vi "hydrolyse_reactor_repetition_check.vi"(10 "#":i32, 11 "Prior Reactor":refnum<vi>) -> (1 "Prior Path":path, 2 "Current Path":path, 3 "Repetition?":bool)   [LabVIEW 2019]
uses:
  lib/libSimulationControl/libSimulationControl.lvlib
panel:
  out "source":path
  out "target":path
  # "*******************************************************************\nBiogas Plant Control\n\nAuthor: Paul Zügel\nGCSC-Frankfurt am Main 2020\n\n*******************************************************************"
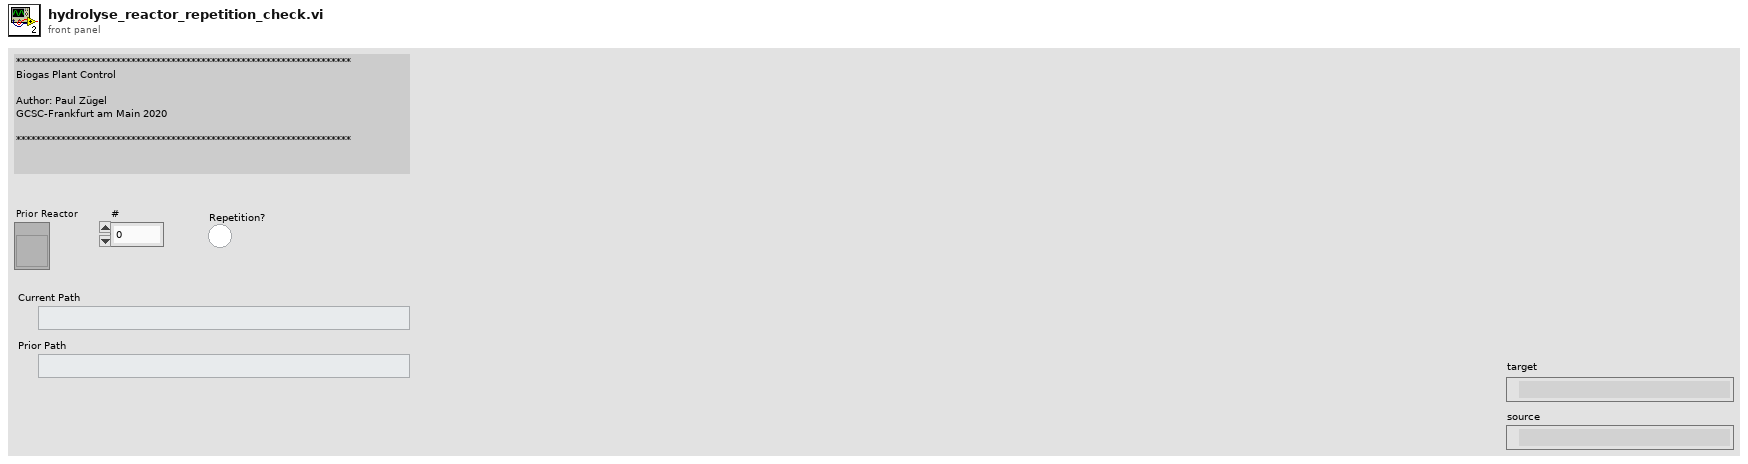
[diagram p1: front panel]
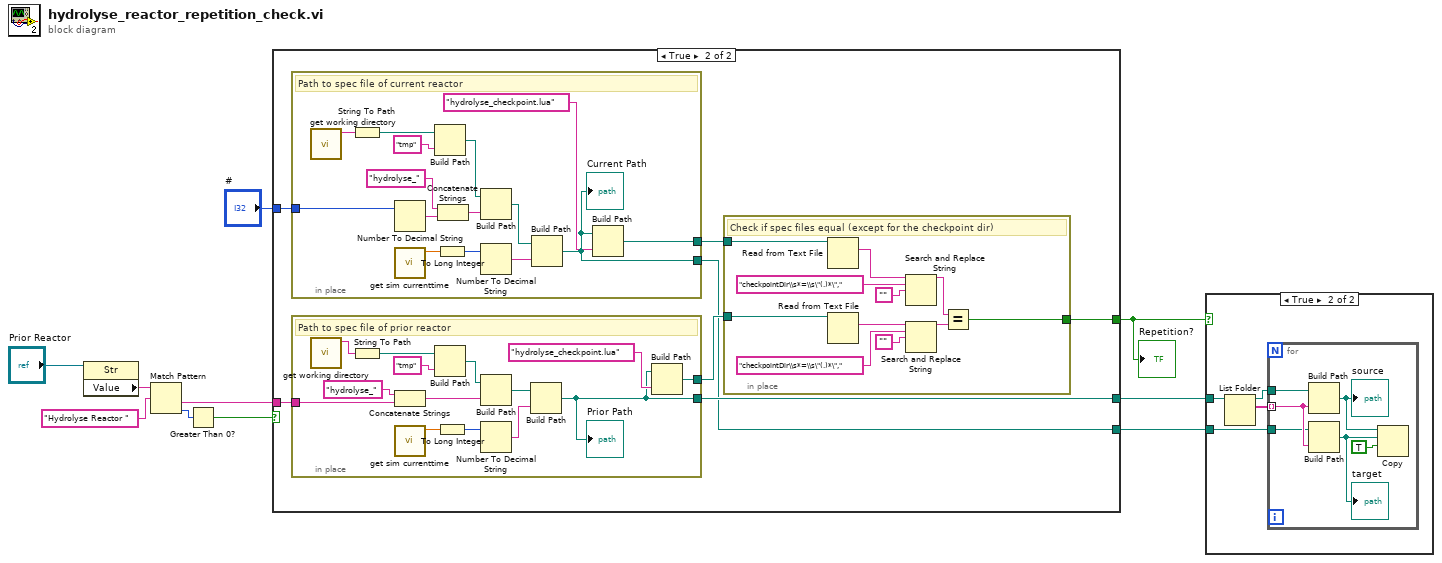
[diagram p0: block diagram]
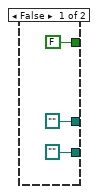
[diagram p3: hidden frame]
diagram:
  n1 = property class="Str"(reference="Prior Reactor") -> ("Value"=w10:string)  [unwired: 1 in, 2 out]
  n2 = Match Pattern(string=w10, regular expression="Hydrolyse Reactor ") -> (after substring=w6:string, offset past match=w8:i32)  [unwired: 1 in, 2 out]
  n3 = Greater Than 0?(x=w8) -> (x > 0?=w7:bool)
  n4 = case shown="True" w7 {
    tunnel: w6 -> [_ w20]
    tunnel: "#" -> [_ w19]
    tunnel: [FALSE w16] -> w3
    tunnel: [path "" w15] -> w2
    tunnel: [path "" w14] -> w1
    frame False {
    }
    frame True {
      n5 = in-place {
        in-place-border: w19 -> [w55]
        in-place-border: [w47] -> w18
        in-place-border: [w46] -> w14
        # "Path to spec file of current reactor"
        n6 = call "get working directory.vi"() -> ("function return"=w52:string)  [unwired: 10 in, 1 out]
        n7 = String To Path(string=w52) -> (path=w58:path)
        n8 = Number To Decimal String(number=w55) -> (decimal integer string=w54:string)  [unwired: 1 in]
        n9 = call "get sim currenttime.vi"() -> ("current_time"=w51:dbl)  [unwired: 10 in, 1 out]
        n10 = Build Path(base path=w58, name or relative path="tmp") -> (appended path=w59:path)
        n11 = To Long Integer(number=w51) -> (32bit integer=w50:i32)
        n12 = Concatenate Strings("hydrolyse_" ("string"), w54) -> (w60:string)
        n13 = Build Path(base path=w59, name or relative path=w60) -> (appended path=w53:path)
        n14 = Number To Decimal String(number=w50) -> (decimal integer string=w49:string)  [unwired: 1 in]
        n15 = Build Path(base path=w53, name or relative path=w49) -> (appended path=w46:path)
        "Current Path" <- w46
        n16 = Build Path(base path=w46, name or relative path="hydrolyse_checkpoint.lua") -> (appended path=w47:path)
      }
      n17 = in-place "In Place Element Structure" {
        in-place-border: w20 -> [w40]
        in-place-border: [w33] -> w17
        in-place-border: [w32] -> w15
        # "Path to spec file of prior reactor"
        n18 = call "get working directory.vi"() -> ("function return"=w35:string)  [unwired: 10 in, 1 out]
        n19 = String To Path(string=w35) -> (path=w43:path)
        n20 = Concatenate Strings("hydrolyse_" ("string"), w40) -> (w45:string)
        n21 = call "get sim currenttime.vi"() -> ("current_time"=w38:dbl)  [unwired: 10 in, 1 out]
        n22 = Build Path(base path=w43, name or relative path="tmp") -> (appended path=w44:path)
        n23 = To Long Integer(number=w38) -> (32bit integer=w37:i32)
        n24 = Build Path(base path=w44, name or relative path=w45) -> (appended path=w39:path)
        n25 = Number To Decimal String(number=w37) -> (decimal integer string=w36:string)  [unwired: 1 in]
        n26 = Build Path(base path=w39, name or relative path=w36) -> (appended path=w32:path)
        "Prior Path" <- w32
        n27 = Build Path(base path=w32, name or relative path="hydrolyse_checkpoint.lua") -> (appended path=w33:path)
      }
      n28 = in-place {
        in-place-border: w18 -> [w31]
        in-place-border: w17 -> [w30]
        in-place-border: [w29] -> w16
        # "Check if spec files equal (except for the checkpoint dir)"
        n29 = Read from Text File(file (use dialog)=w31) -> (text=w28:string)  [unwired: 3 in, 3 out]
        n30 = Read from Text File(file (use dialog)=w30) -> (text=w25:string)  [unwired: 3 in, 3 out]
        n31 = Search and Replace String(input string=w28, search string="checkpointDir\\s*=\\s\"(.)*\",", replace string="") -> (result string=w21:string)  [unwired: 5 in, 3 out]
        n32 = Search and Replace String(input string=w25, search string="checkpointDir\\s*=\\s\"(.)*\",", replace string="") -> (result string=w22:string)  [unwired: 5 in, 3 out]
        n33 = Equal?(x=w21, y=w22) -> (x = y?=w29:bool)
      }
    }
  }
  "Repetition?" <- w3
  n34 = case shown="True" w3 {
    tunnel: w2 -> [_ w62]
    tunnel: w1 -> [_ w61]
    frame False {
    }
    frame True {
      n35 = List Folder(path=w62) -> (path out=w63:path, filenames=w64:string[])  [unwired: 3 in, 2 out]
      n36 = for {
        tunnel: w64 -> [w69] mode=indexing
        tunnel: w63 -> [w70]
        tunnel: w61 -> [w65]
        n37 = Build Path(base path=w70, name or relative path=w69) -> (appended path=w67:path)
        "source" <- w67
        n38 = Build Path(base path=w65, name or relative path=w69) -> (appended path=w66:path)
        "target" <- w66
        n39 = Copy(9:TRUE ("overwrite (F)"), 10:w66, 11:w67) -> ()  [unwired: 2 in, 3 out]
      }
    }
  }
